vi "test Copy Equal Size.vi"(8 "error in (no error)":errorcluster, 11 "TestCase in":refnum<class "Data Manipulation Tests.lvclass">) -> (0 "error out":errorcluster, 3 "TestCase out":refnum<class "Data Manipulation Tests.lvclass">)   [LabVIEW 2017, in "Pointer Tests.lvlib" / "Data Manipulation Tests.lvclass"]
uses:
  Data Manipulation Tests.lvclass
  Source/Classes/Pointer/Write 1D I32.vi
  <vilib>/addons/_JKI Toolkits/VI Tester/TestCase.llb/TestCase.lvclass
  Source/Classes/Pointer/Pointer.lvclass
  C:/Program Files (x86)/National Instruments/LabVIEW 2017/vi.lib/addons/_JKI Toolkits/VI Tester/TestCase.llb/TestCase.lvclass
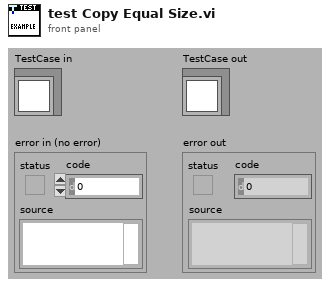
[diagram p1: front panel]
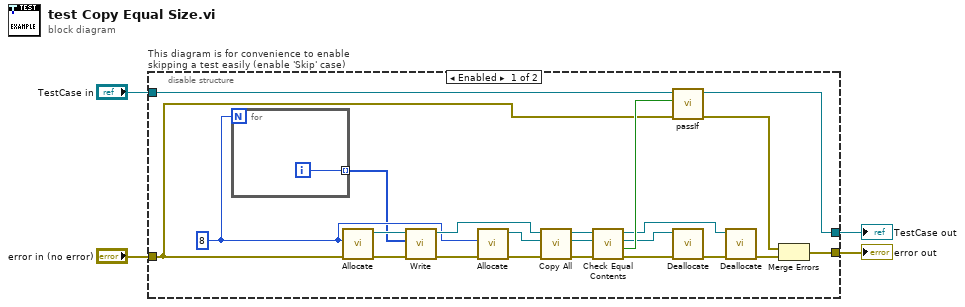
[diagram p0: block diagram]
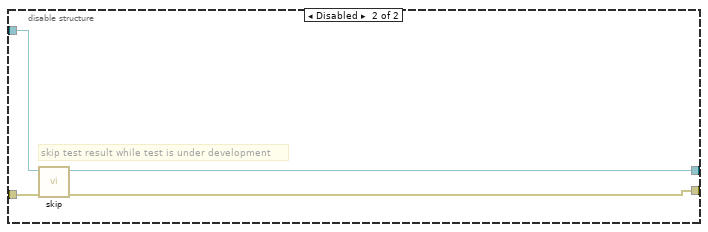
[diagram p2: hidden frame]
diagram:
  n1 = disable-structure "This diagram is for convenience to enable skipping a test easily (enable 'Skip' case)" shown="Enabled" {
    disable-tunnel: "TestCase in" -> [w19 w31]
    disable-tunnel: [w18 w29] -> w1
    disable-tunnel: [w13 w30] -> w3
    disable-tunnel: "error in (no error)" -> [w8 w28]
    frame Enabled {
      w24 = u64 8 ("count (1)")
      n2 = for {
        N: w24 -> [_]
        tunnel: [w27] -> w5 mode=indexing
        i -> [w27]
      }
      n3 = call "Allocate.vi"("error in (no error)"=w8, "size"=w24) -> ("error out"=w16:errorcluster, "Pointer out"=w26:refnum<class "Pointer.lvclass">)  [unwired: 8 in]
      n4 = call-poly "Write.vi"("error in (no error)"=w16, "buffer in"=w5, "Pointer in"=w26) -> ("error out"=w15:errorcluster, "Pointer out"=w25:refnum<class "Pointer.lvclass">)  [unwired: 5 in, 2 out]
      n5 = call "Allocate.vi"("error in (no error)"=w15, "size"=w24) -> ("error out"=w14:errorcluster, "Pointer out"=w23:refnum<class "Pointer.lvclass">)  [unwired: 8 in]
      n6 = call "Copy All.vi"("error in (no error)"=w14, "dst Pointer in"=w23, "src Pointer in"=w25) -> ("error out"=w11:errorcluster, "dst Pointer out"=w21:refnum<class "Pointer.lvclass">, "src Pointer out"=w22:refnum<class "Pointer.lvclass">)  [unwired: 6 in]
      n7 = call "Check Equal Contents.vi"("error in (no error)"=w11, "pointer y"=w21, "pointer x"=w22) -> ("error out"=w12:errorcluster, "equal contents?"=w17:bool, "pointer y"=w9:refnum<class "Pointer.lvclass">, "pointer x"=w6:refnum<class "Pointer.lvclass">)  [unwired: 5 in]
      n8 = call-dynamic "passIf.vi"("error in (no error)"=w8, "pass"=w17, "TestCase in"=w19) -> ("error out"=w20:errorcluster, "TestCase out"=w18:refnum<class "Data Manipulation Tests.lvclass">)  [unwired: 7 in]
      n9 = call "Deallocate.vi"("error in (no error)"=w12, "Pointer in"=w9) -> ("error out"=w10:errorcluster)  [unwired: 8 in, 1 out]
      n10 = call "Deallocate.vi"("error in (no error)"=w10, "Pointer in"=w6) -> ("error out"=w7:errorcluster)  [unwired: 8 in, 1 out]
      n11 = Merge Errors(w20, w7) -> (w13:errorcluster)
    }
    frame Disabled {
      # "skip test result while test is under development"
      n12 = call <vilib>:"skip.vi"("error in (no error)"=w28, "TestCase in"=w31) -> ("error out"=w30:errorcluster, "TestCase out"=w29:refnum<class "Data Manipulation Tests.lvclass">)  [unwired: 8 in]
    }
  }
  "error out" <- w3
  "TestCase out" <- w1
